vi "Put pixels.vi"(0 "Xc":i32, 5 "Yc":i32, 7 "X":i32, 9 "Y":i32, 11 "error in (no error)":errorcluster) -> (4 "Pixels":cluster{"X":i32, "Y":i32}[](array[cluster]), 15 "error out":errorcluster)   [LabVIEW 2017]
doc: "To get the pixels from other octants."
panel:
  in  "Coords":cluster{"X":i32, "Y":i32}
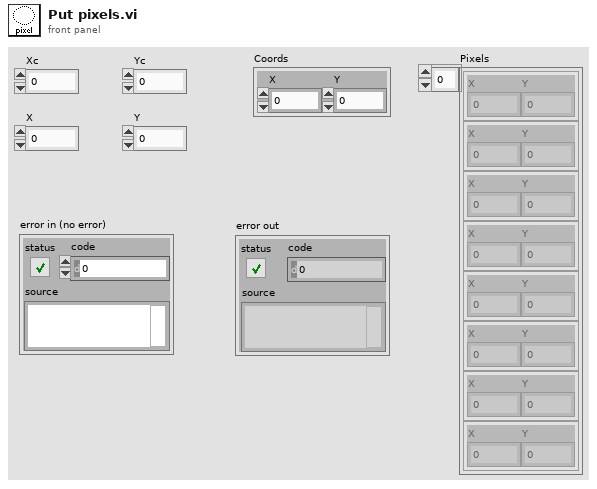
[diagram p1: front panel]
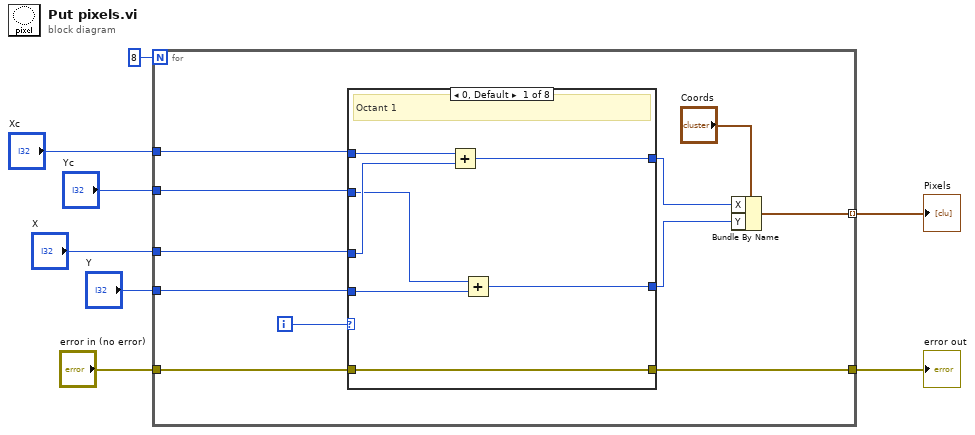
[diagram p0: block diagram]
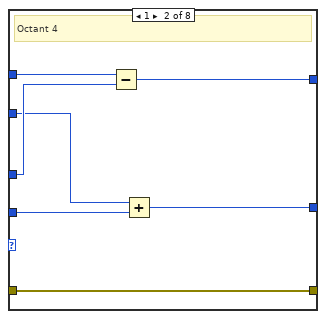
[diagram p2: hidden frame]
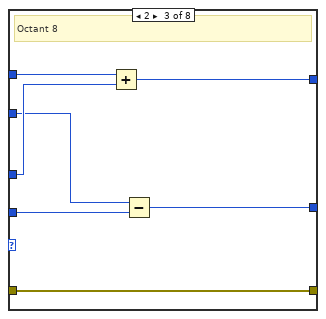
[diagram p3: hidden frame]
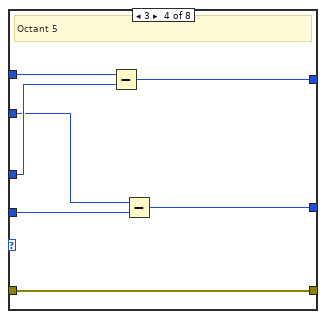
[diagram p4: hidden frame]
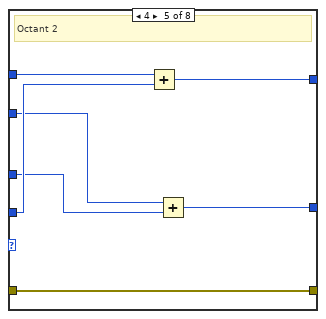
[diagram p5: hidden frame]
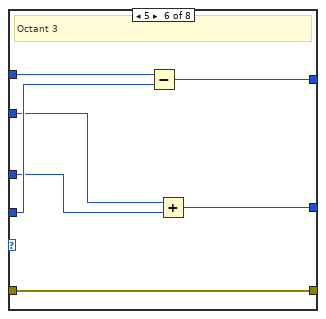
[diagram p6: hidden frame]
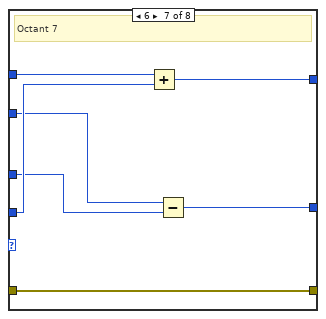
[diagram p7: hidden frame]
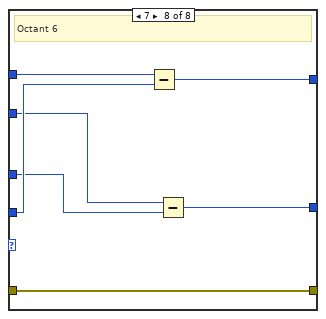
[diagram p8: hidden frame]
diagram:
  n1 = for {
    N: 8 -> [_]
    tunnel: [w15] -> w4 mode=indexing
    tunnel: "Yc" -> [w14]
    tunnel: "Xc" -> [w13]
    tunnel: "Y" -> [w12]
    tunnel: "X" -> [w11]
    tunnel: "error in (no error)" -> [w10]
    tunnel: [w9] -> w1
    i -> [w19]
    n2 = case shown="0, Default" w19 {
      tunnel: w11 -> [w25 w32 w39 w46 w51 w58 w65 w72]
      tunnel: w12 -> [w23 w30 w37 w44 w53 w60 w67 w74]
      tunnel: w13 -> [w26 w33 w40 w47 w54 w61 w68 w75]
      tunnel: w14 -> [w24 w31 w38 w45 w52 w59 w66 w73]
      tunnel: [w22 w29 w36 w43 w49 w56 w63 w70] -> w18
      tunnel: [w21 w28 w35 w42 w50 w57 w64 w71] -> w17
      tunnel: w10 -> [w20 w27 w34 w41 w48 w55 w62 w69]
      tunnel: [w20 w27 w34 w41 w48 w55 w62 w69] -> w9
      frame 0, Default {
        # "Octant 1"
        n3 = Add(x=w26, y=w25) -> (x+y=w22:i32)
        n4 = Add(x=w24, y=w23) -> (x+y=w21:i32)
      }
      frame 1 {
        # "Octant 4"
        n5 = Subtract(x=w33, y=w32) -> (x-y=w29:i32)
        n6 = Add(x=w31, y=w30) -> (x+y=w28:i32)
      }
      frame 2 {
        # "Octant 8"
        n7 = Add(x=w40, y=w39) -> (x+y=w36:i32)
        n8 = Subtract(x=w38, y=w37) -> (x-y=w35:i32)
      }
      frame 3 {
        # "Octant 5"
        n9 = Subtract(x=w47, y=w46) -> (x-y=w43:i32)
        n10 = Subtract(x=w45, y=w44) -> (x-y=w42:i32)
      }
      frame 4 {
        # "Octant 2"
        n11 = Add(x=w54, y=w53) -> (x+y=w49:i32)
        n12 = Add(x=w52, y=w51) -> (x+y=w50:i32)
      }
      frame 5 {
        # "Octant 3"
        n13 = Subtract(x=w61, y=w60) -> (x-y=w56:i32)
        n14 = Add(x=w59, y=w58) -> (x+y=w57:i32)
      }
      frame 6 {
        # "Octant 7"
        n15 = Add(x=w68, y=w67) -> (x+y=w63:i32)
        n16 = Subtract(x=w66, y=w65) -> (x-y=w64:i32)
      }
      frame 7 {
        # "Octant 6"
        n17 = Subtract(x=w75, y=w74) -> (x-y=w70:i32)
        n18 = Subtract(x=w73, y=w72) -> (x-y=w71:i32)
      }
    }
    n19 = Bundle By Name(cluster="Coords", "X"=w18, "Y"=w17) -> (w15:cluster{"X":i32, "Y":i32})
  }
  "Pixels" <- w4
  "error out" <- w1
